vi "fgv_error-2.vi"(7 "cmd":enum16{"init", "read", "write"}(ring), 8 "error in":errorcluster, 11 "Error cluster":T2={"AGV"=0, "AGV Estop"=0, "Obstacle"=0, "Heading"=0, "Waypt"=0, "GNSS"=0, "VLP16"=0, "Cam"=0, "RPLidar"=2, "Joystick"=2}) -> (0 "error out":errorcluster, 3 "Error cluster out":T2={"AGV"=0, "AGV Estop"=0, "Obstacle"=0, "Heading"=0, "Waypt"=0, "GNSS"=0, "VLP16"=0, "Cam"=0, "RPLidar"=2, "Joystick"=2})   [LabVIEW 2019]
uses:
  Ctrl/status.ctl
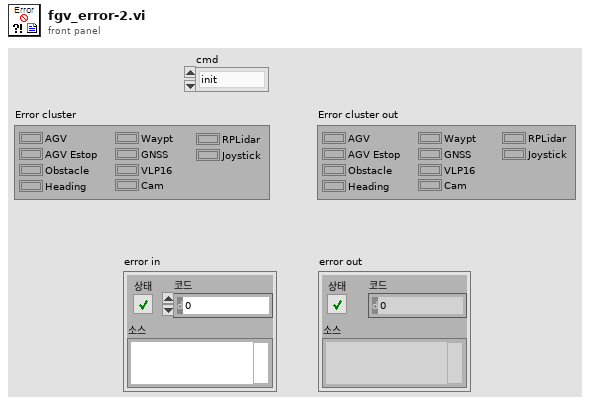
[diagram p1: front panel]
types:
  T1 = typedef "status.ctl" = u16
  T2 = cluster{"AGV":T1, "AGV Estop":T1, "Obstacle":T1, "Heading":T1, "Waypt":T1, "GNSS":T1, "VLP16":T1, "Cam":T1, "RPLidar":T1, "Joystick":T1}
  T3 = cluster{"AGV":T1, "AGV Estop":T1, "Obstacle":T1, "Heading":T1, "Waypt":T1, "GNSS":T1, "VLP16":T1, "AGV 2":T1, "AGV 3":T1, "AGV 4":T1}
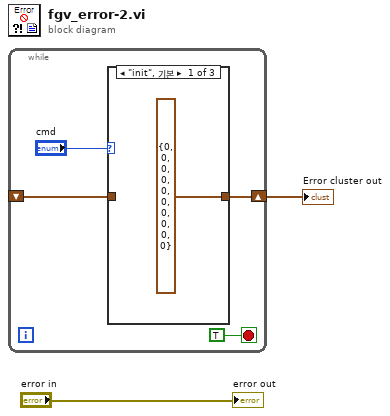
[diagram p0: block diagram]
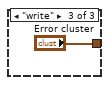
[diagram p3: hidden frame]
diagram:
  n1 = while {
    shift-right: [w4] -> w1
    shift-left: _ -> [w3]
    stop <- TRUE stop-if-true
    n2 = case shown="\"init\", 기본" "cmd" {
      tunnel: [T3 {"AGV"=0, "AGV Estop"=0, "Obstacle"=0, "Heading"=0, "Waypt"=0, "GNSS"=0, "VLP16"=0, "AGV 2"=0, "AGV 3"=0, "AGV 4"=0} ("Error cluster") w8 "Error cluster"] -> w4
      tunnel: w3 -> [_ w8 _]
      frame "init", Default {
      }
      frame "read" {
      }
      frame "write" {
      }
    }
  }
  "Error cluster out" <- w1
  "error out" <- "error in"
